vi "AddSyncSig.vi"(8 "error in":errorcluster, 10 "inputData":cdb[](array[numeric]), 11 "Path In":path) -> (0 "error out":errorcluster, 2 "out_data":cdb[](array[numeric]), 3 "Path Out":path)   [LabVIEW 2015]
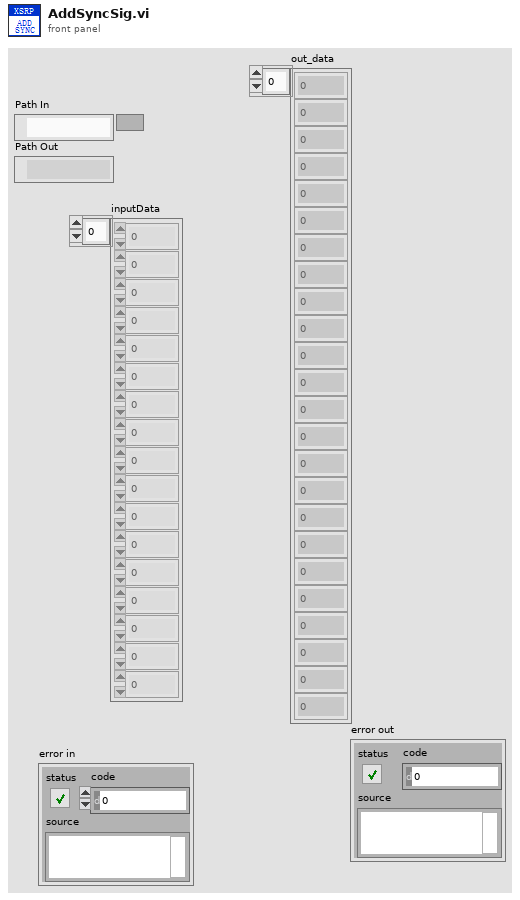
[diagram p1: front panel]
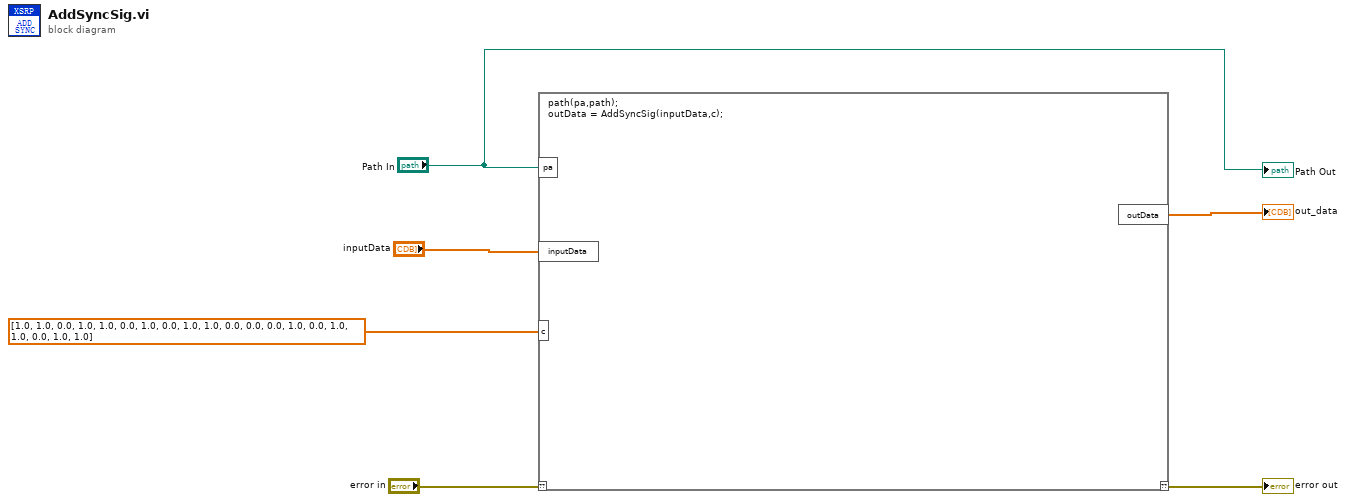
[diagram p0: block diagram]
diagram:
  n1 = script code="path(pa,path);\noutData = AddSyncSig(inputData,c);"("??"="error in", "pa"="Path In", "inputData"="inputData", "c"=dbl[] [1.0, 1.0, 0.0, 1.0, 1.0, 0.0, 1.0, 0.0, 1.0, 1.0, 0.0, 0.0, 0.0, 1.0, 0.0, 1.0, 1.0, 0.0, 1.0, 1.0]) -> ("??"=→"error out":errorcluster, "outData"=→"out_data":cdb[])
  "Path Out" <- "Path In"
